vi "Concatenate Submodule Name.vi"(10 "Module Name":string, 11 "Group Name":string) -> (3 "Submodule Name":string)   [LabVIEW 2017, in "Communicable State Machine.lvlib"]
doc: "Constructs a submodule name.\n\n-- <b>Controls</b> --\n- <b>CSM Name</b>: CSM module name.\n- <b>Name</b>: Name to append to the CSM module name.\n\n-- <b>Indicators</b> --\n- <b>Submodule Name</b>: Returns the concatenated submodule name."
uses:
  Communicable State Machine.lvlib
  _Shared/CSM Shared.lvlib
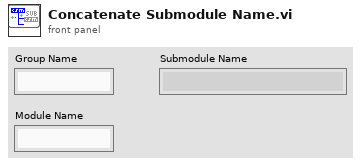
[diagram p1: front panel]
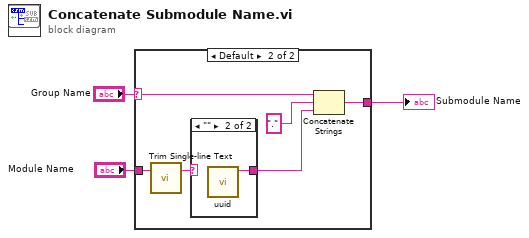
[diagram p0: block diagram]
diagram:
  n1 = case shown="Default" "Group Name" {
    selector: "Group Name" -> [_ w8]
    tunnel: [w4 w10] -> w3
    tunnel: "Module Name" -> [w4 w7]
    frame "" {
    }
    frame Default {
      n2 = call "Trim Single-line Text.vi"("single-line text"=w7) -> ("trimed text"=w5:string)  [unwired: 2 in]
      n3 = case shown="\"\"" w5 {
        selector: w5 -> [w11 _]
        tunnel: [w11 w12] -> w6
        frame "False", Default {
        }
        frame "" {
          n4 = call "uuid.vi"() -> ("UUID"=w12:string)  [unwired: 11 in]
        }
      }
      n5 = Concatenate Strings(w8, "." ("string"), w6) -> (w10:string)
    }
  }
  "Submodule Name" <- w3
